vi "Panel close.vi"(2 "error in":errorcluster, 3 "This VI":refnum<vi>) -> (0 "error out":errorcluster)   [LabVIEW 2010]
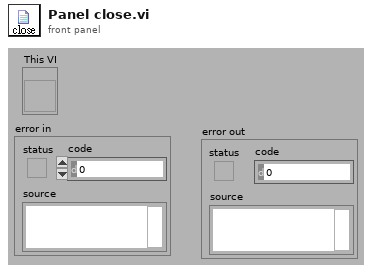
[diagram p1: front panel]
types:
  T1 = enum32{"invalid app kind", "Development System", "Run Time System", "Student Edition", "Embedded LabVIEW", "Evaluation", "Custom"}
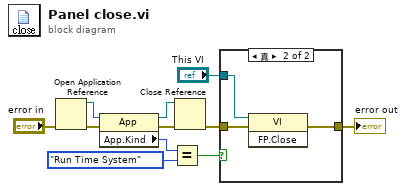
[diagram p0: block diagram]
diagram:
  n1 = Open Application Reference(8:"error in") -> (0:w7:errorcluster, 3:w6:refnum<vi>)  [unwired: 3 in]
  n2 = property class="App"(reference=w6, error in=w7) -> (reference out=w4:refnum<vi>, error out=w3:errorcluster, "App.Kind"=w9:T1)
  n3 = Equal?(x=w9, y=T1."Run Time System" ("Application:Kind")) -> (x = y?=w11:bool)
  n4 = Close Reference(reference=w4, error in (no error)=w3) -> (error out=w2:errorcluster)
  n5 = case shown="真" w11 {
    tunnel: w2 -> [w12 w15]
    tunnel: "This VI" -> [_ w14]
    tunnel: [w12 w13] -> w1
    frame False {
    }
    frame True {
      n6 = invoke class="VI" method="FP.Close"(reference=w14, error in=w15) -> (error out=w13:errorcluster)  [unwired: 1 in, 2 out]
    }
  }
  "error out" <- w1
